vi "Handle Graph Data.vi"(8 "error in":errorcluster, 9 "graph in":dbl[][](graph), 10 "plotNames in":string[](array[string]), 11 "clsData":T1) -> (0 "error out":errorcluster, 1 "graph out":dbl[][](graph), 2 "plotNames out":string[](array[string]))   [LabVIEW 2013]
uses:
  controls/clsData.ctl
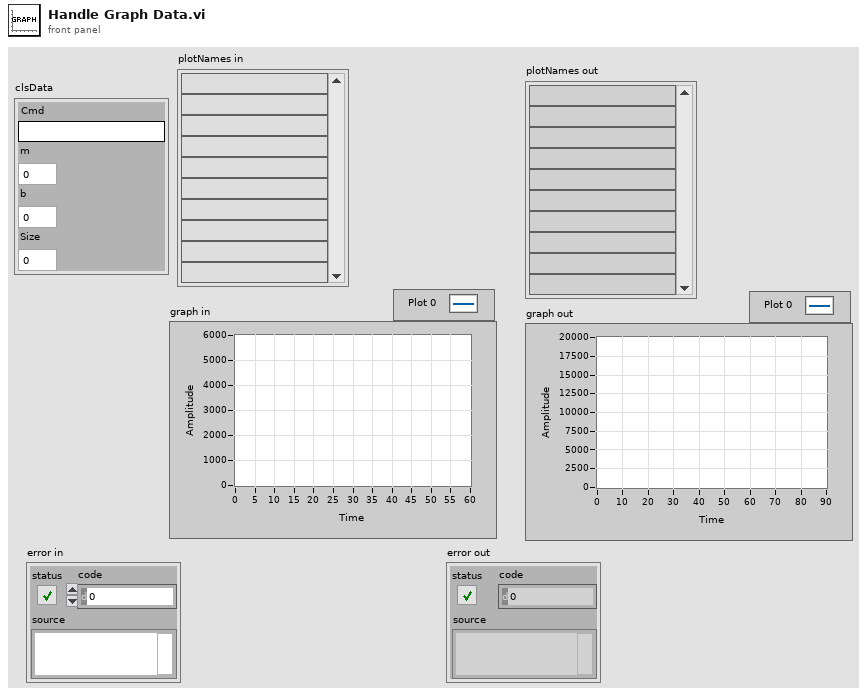
[diagram p1: front panel]
types:
  T1 = typedef "clsData.ctl" = cluster{"Cmd":string, "m":dbl, "b":dbl, "Size":u32}
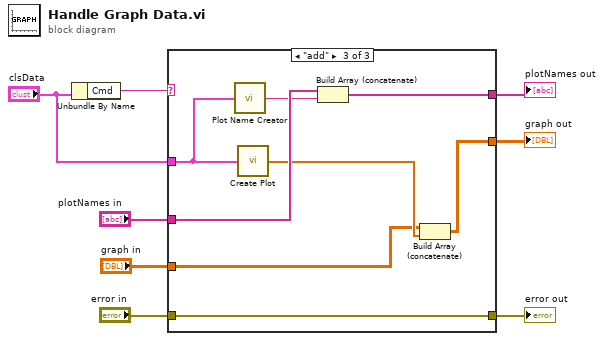
[diagram p0: block diagram]
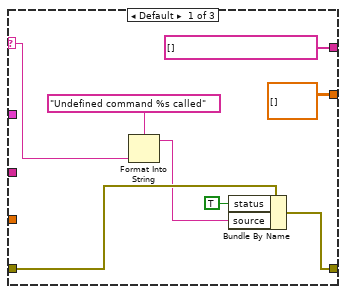
[diagram p2: hidden frame]
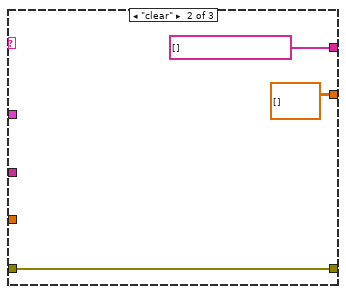
[diagram p3: hidden frame]
diagram:
  n1 = Unbundle By Name("clsData") -> ("Cmd"=w8:string)
  n2 = case shown="\"add\"" w8 {
    selector: w8 -> [w12 _ _]
    tunnel: [dbl[][] [] ("graph in") dbl[][] [] ("graph in") w20] -> w1
    tunnel: [string[] [] ("plotNames out") string[] [] ("plotNames out") w24] -> w7
    tunnel: "clsData" -> [_ _ w27]
    tunnel: "plotNames in" -> [_ _ w26]
    tunnel: "error in" -> [w15 w18 w23]
    tunnel: [w10 w18 w23] -> w3
    tunnel: "graph in" -> [_ _ w21]
    frame Default {
      n3 = Format Into String(format string="Undefined command %s called" ("source"), w12) -> (resulting string=w11:string)  [unwired: 2 in, 1 out]
      n4 = Bundle By Name(cluster=w15, "status"=TRUE, "source"=w11) -> (w10:errorcluster)
    }
    frame "clear" {
    }
    frame "add" {
      n5 = call "Plot Name Creator.vi"("clsData"=w27) -> ("plotName"=w25:string)
      n6 = call "Create Plot.vi"("clsData"=w27) -> ("Plot"=w22:dbl[])
      n7 = Build Array (concatenate)(w26, w25) -> (w24:string[])
      n8 = Build Array (concatenate)(w21, w22) -> (w20:dbl[][])
    }
  }
  "error out" <- w3
  "graph out" <- w1
  "plotNames out" <- w7
